vi "ServoRefNum_Simulation_Global.vi"(0 "menu":enum16{"set", "get", "delete"}(ring)=enum."get", 7 "PWM Channel":T1, 9 "Servo Set":refnum<class "Parallax Standard Servo.lvclass">, 11 "error in (no error)":errorcluster) -> (10 "Servo Get":refnum<class "Parallax Standard Servo.lvclass">, 15 "error out":errorcluster)   [LabVIEW 2017]
doc: "Sets a reference into a registry, gets a reference from a registry, or deletes a reference from a registry. The reference is accessed by name, and can be given any unique name.\n\nThis software is licensed. Open the labview\\readme\\WPI Robotics Library Open Source License.txt file for more information."
uses:
  <instrlib>/Parallax Standard Servo/HAIOL/Parallax Standard Servo.lvclass
  <vilib>/Rock Robotics/SystemInterfaces/DIO/FPGA_DIOPWMChannel.ctl
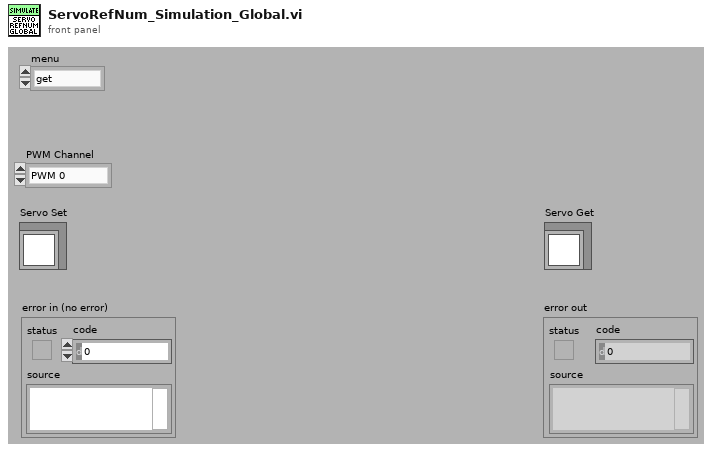
[diagram p1: front panel]
types:
  T1 = typedef "FPGA_DIOPWMChannel.ctl" = enum8{"PWM 0", "PWM 1", "PWM 2", "PWM 3", "PWM 4", "PWM 5", "PWM 6", "PWM 7", "PWM 8", "PWM 9", "PWM MXP 0", "PWM MXP 1", "PWM MXP 2", "PWM MXP 3", "PWM MXP 4", "PWM MXP 5", "PWM MXP 6", "PWM MXP 7", "PWM MXP 8", "PWM MXP 9", "Invalid"}
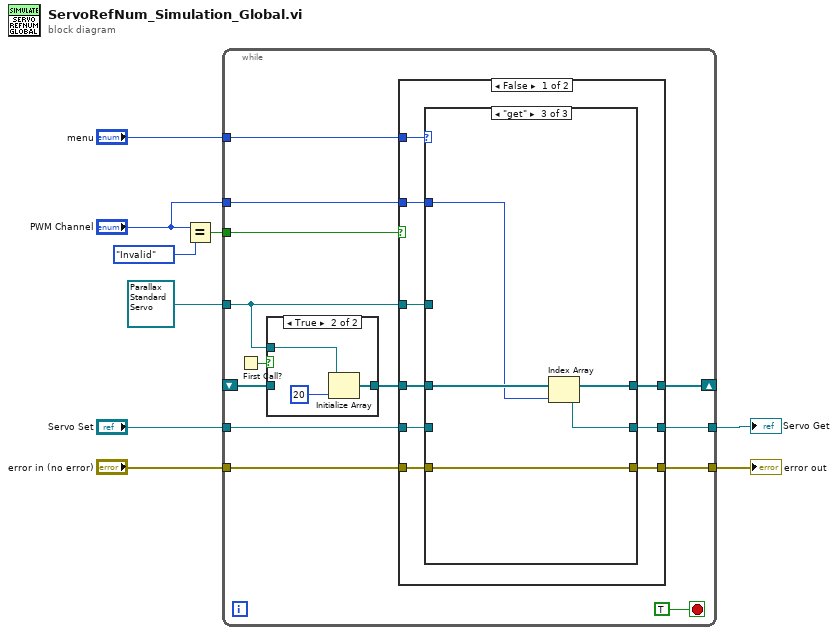
[diagram p0: block diagram]
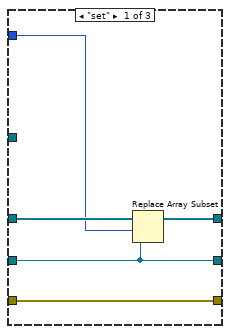
[diagram p2: hidden frame]
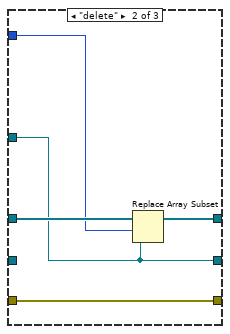
[diagram p3: hidden frame]
diagram:
  n1 = Equal?(x="PWM Channel", y=FPGA_DIOPWMChannel."Invalid" ("PWM Channel")) -> (x = y?=w6:bool)
  n2 = while {
    tunnel: "Servo Set" -> [w22]
    tunnel: "error in (no error)" -> [w18]
    shift-right: [w21] -> _
    shift-left: _ -> [w13]
    tunnel: [w20] -> w4
    tunnel: "menu" -> [w19]
    tunnel: [w17] -> w8
    tunnel: "PWM Channel" -> [w12]
    tunnel: w6 -> [w11]
    tunnel: refnum<class "Parallax Standard Servo.lvclass"> refnum ("Servo Get") -> [w10]
    stop <- TRUE stop-if-true
    n3 = First Call?() -> (First Call?: T/F=w15:bool)
    n4 = case shown="True" w15 {
      tunnel: [w49 w51] -> w14
      tunnel: w13 -> [w49 _]
      tunnel: w10 -> [_ w50]
      frame False {
      }
      frame True {
        n5 = Initialize Array(w50, 20 ("dimension size")) -> (w51:refnum<class "Parallax Standard Servo.lvclass">[])
      }
    }
    n6 = case shown="False" w11 {
      tunnel: w22 -> [w31 _]
      tunnel: [w30 w48] -> w21
      tunnel: [w29 w46] -> w20
      tunnel: w19 -> [w28 _]
      tunnel: w18 -> [w27 w47]
      tunnel: [w26 w47] -> w17
      tunnel: w14 -> [w25 w48]
      tunnel: w12 -> [w24 _]
      tunnel: w10 -> [w23 w46]
      frame False {
        n7 = case shown="\"get\"" w28 {
          tunnel: w31 -> [w34 _ _]
          tunnel: [w35 w40 w45] -> w30
          tunnel: w25 -> [w36 w41 w45]
          tunnel: [w34 w37 w42] -> w29
          tunnel: [w33 w39 w44] -> w26
          tunnel: w27 -> [w33 w39 w44]
          tunnel: w24 -> [w32 w38 w43]
          tunnel: w23 -> [_ w37 _]
          frame "set" {
            n8 = Replace Array Subset(array=w36, new element=w34, index=w32) -> (w35:refnum<class "Parallax Standard Servo.lvclass">[])
          }
          frame "delete" {
            n9 = Replace Array Subset(array=w41, new element=w37, index=w38) -> (w40:refnum<class "Parallax Standard Servo.lvclass">[])
          }
          frame "get" {
            n10 = Index Array(array=w45, index=w43) -> (element=w42:refnum<class "Parallax Standard Servo.lvclass">)
          }
        }
      }
      frame True {
        # "Do nothing if PWM channel is Invalid."
      }
    }
  }
  "error out" <- w8
  "Servo Get" <- w4
